vi "GEN_CulArray.vi"(8 "Max Values":i32, 9 "Data_Cluster":T1={"Value"=0.0, "GUI Data Cluster"={"S11"=FALSE, "S21"=FALSE, "S12"=FALSE, "S22"=FALSE, "S11Meas"=enum."Log-magnitude (dB)", "S21Meas"=enum."Log-magnitude (dB)", "S12Meas"=enum."Log-magnitude (dB)", "S22Meas"=enum."Log-magnitude (dB)"}, "Timing"={"Last Operation"=0.0, "Stop @ T/B"=FALSE, "Last Temp"=0.0, "Last Mag"=0.0, "Ramp Param"={"End T (K)"=0.0, "Delta T (K)"=0.0, "End B (T)"=0.0, "Delta B (T)"=0.0}, "LastOp?"=FALSE}, "Measurements"=[], "Hardware"={"VNA TCP Con"=refnum, "VNA TCP Port"=5025, "Global T VAR"="", "Global B VAR"=""}, "Operation"={"Operation Mode"=enum."Logging", "Log Folder"=path "", "Measure Mode"=enum."Deltat"}}) -> (1 "Data_Cluster Out":T1={"Value"=0.0, "GUI Data Cluster"={"S11"=FALSE, "S21"=FALSE, "S12"=FALSE, "S22"=FALSE, "S11Meas"=enum."Log-magnitude (dB)", "S21Meas"=enum."Log-magnitude (dB)", "S12Meas"=enum."Log-magnitude (dB)", "S22Meas"=enum."Log-magnitude (dB)"}, "Timing"={"Last Operation"=0.0, "Stop @ T/B"=FALSE, "Last Temp"=0.0, "Last Mag"=0.0, "Ramp Param"={"End T (K)"=0.0, "Delta T (K)"=0.0, "End B (T)"=0.0, "Delta B (T)"=0.0}, "LastOp?"=FALSE}, "Measurements"=[], "Hardware"={"VNA TCP Con"=refnum, "VNA TCP Port"=5025, "Global T VAR"="", "Global B VAR"=""}, "Operation"={"Operation Mode"=enum."Logging", "Log Folder"=path "", "Measure Mode"=enum."Deltat"}})   [LabVIEW 2021]
uses:
  Data_Cluster.ctl
  Measurement_Cluster.ctl
  Mode_Enum.ctl
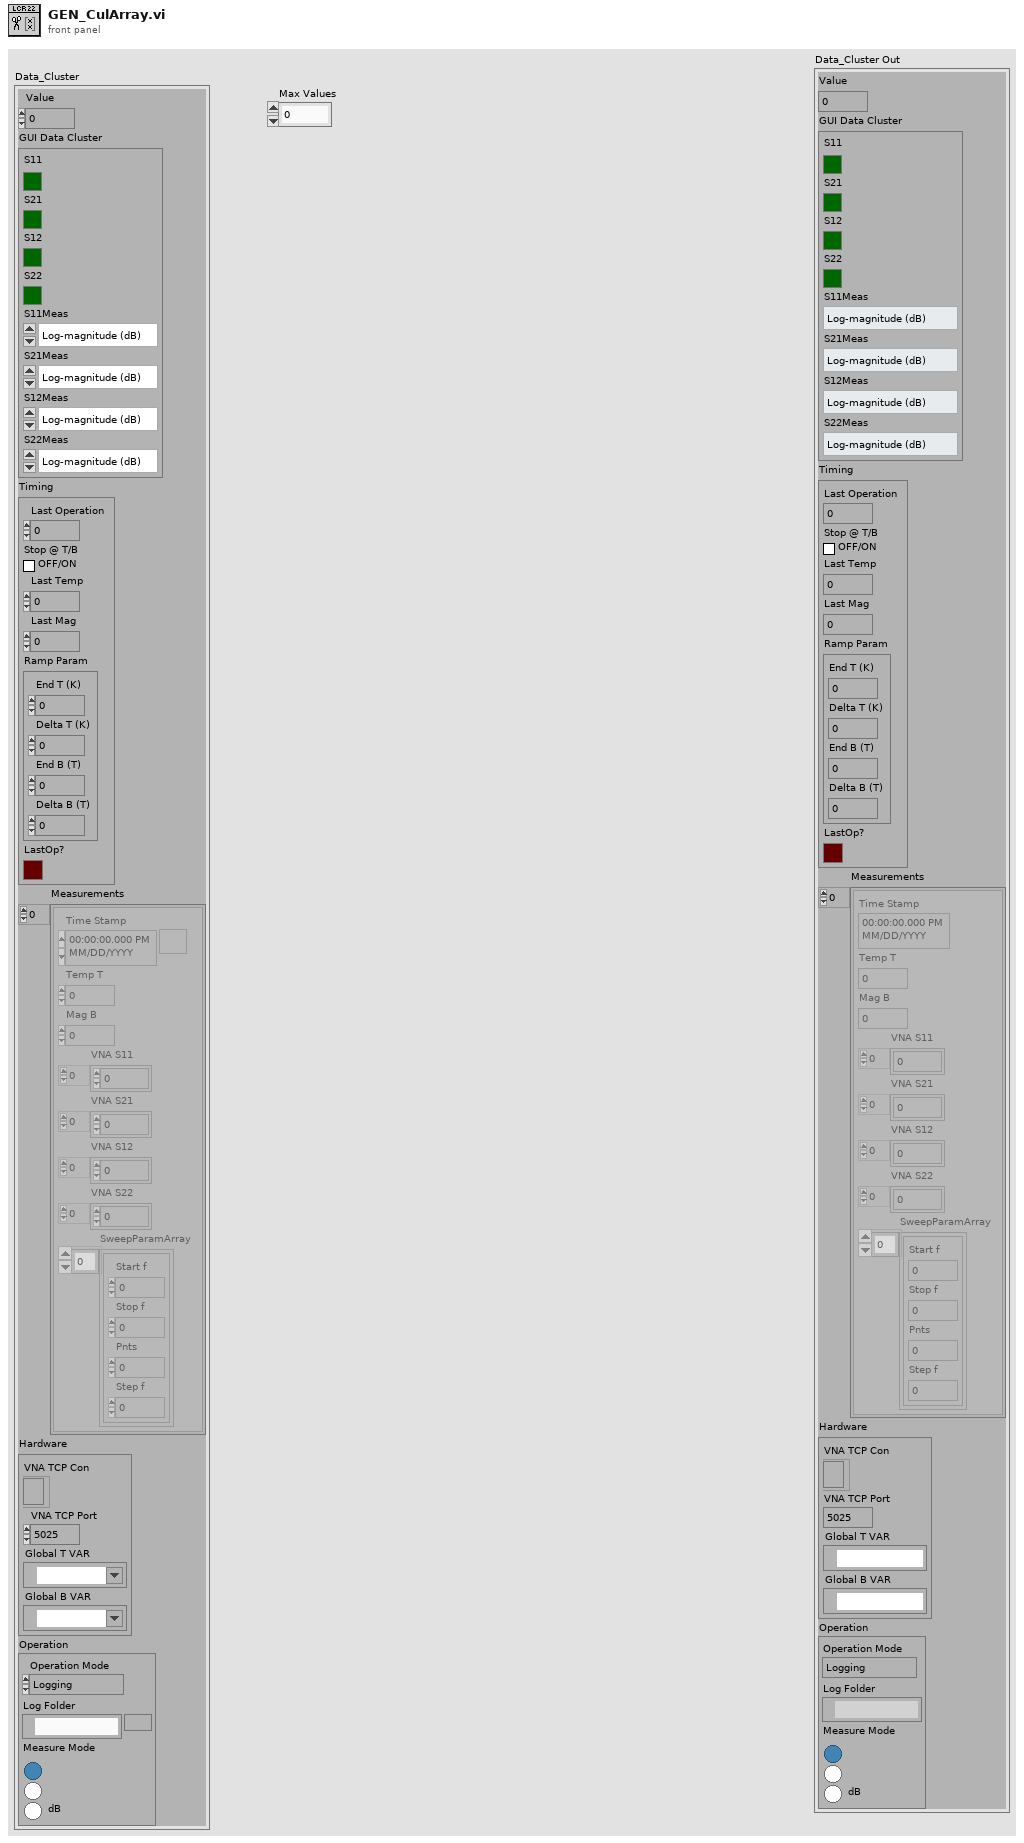
[diagram p1: front panel]
types:
  T1 = typedef "Data_Cluster.ctl" = cluster{"Value":dbl, "GUI Data Cluster":cluster{"S11":bool, "S21":bool, "S12":bool, "S22":bool, "S11Meas":enum16{"Log-magnitude (dB)", "Linear magnitude", "Phase (deg)", "Time Domain", "Real", "Imaginary", "Group Delay", "Polarlinear"}, "S21Meas":enum16{"Log-magnitude (dB)", "Linear magnitude", "Phase (deg)", "Time Domain", "Real", "Imaginary", "Group Delay", "Polarlinear"}, "S12Meas":enum16{"Log-magnitude (dB)", "Linear magnitude", "Phase (deg)", "Time Domain", "Real", "Imaginary", "Group Delay", "Polarlinear"}, "S22Meas":enum16{"Log-magnitude (dB)", "Linear magnitude", "Phase (deg)", "Time Domain", "Real", "Imaginary", "Group Delay", "Polarlinear"}}, "Timing":cluster{"Last Operation":dbl, "Stop @ T/B":bool, "Last Temp":dbl, "Last Mag":dbl, "Ramp Param":cluster{"End T (K)":dbl, "Delta T (K)":dbl, "End B (T)":dbl, "Delta B (T)":dbl}, "LastOp?":bool}, "Measurements":T2[], "Hardware":cluster{"VNA TCP Con":refnum<k5>, "VNA TCP Port":i32, "Global T VAR":refnum<k21>, "Global B VAR":refnum<k21>}, "Operation":cluster{"Operation Mode":T3, "Log Folder":path, "Measure Mode":enum32{"Deltat", "DeltaT", "dB"}}}
  T2 = typedef "Measurement_Cluster.ctl" = cluster{"Time Stamp":timestamp, "Temp T":dbl, "Mag B":dbl, "VNA S11":dbl[], "VNA S21":dbl[], "VNA S12":dbl[], "VNA S22":dbl[], "SweepParamArray":cluster{"Start f":dbl, "Stop f":dbl, "Pnts":i32, "Step f":dbl}[]}
  T3 = typedef "Mode_Enum.ctl" = enum16{"Logging", "Idle-Off", "Idle"}
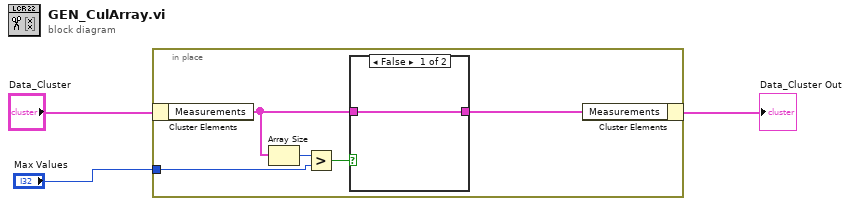
[diagram p0: block diagram]
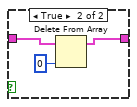
[diagram p2: hidden frame]
diagram:
  n1 = in-place {
    in-place-border: "Max Values" -> [w7]
    n2 = in-place-cluster #1("Data_Cluster") -> ("Measurements"=w5:T2[])
    n3 = Array Size(array=w5) -> (size(s)=w8:i32)
    n4 = Greater?(x=w8, y=w7) -> (0:w6:bool)
    n5 = case shown="False" w6 {
      tunnel: w5 -> [w9 w12]
      tunnel: [w9 w11] -> w4
      frame False {
      }
      frame True {
        n6 = Delete From Array(array=w12, index=0) -> (array with subset deleted=w11:T2[])  [unwired: 1 in, 1 out]
      }
    }
    n7 = in-place-cluster #1("Measurements"=w4) -> (→"Data_Cluster Out":T1)
  }
